vi "Act_LabView3_Task1_jones6sv.vi"() -> ()   [LabVIEW 2016]
uses:
  <vilib>/express/express arith-compare/Formula/XNode/ExpressFormulaBlockNode.xnode
panel:
  out "Numeric":dbl
  in  "Upper limit":dbl
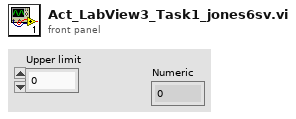
[diagram p1: front panel]
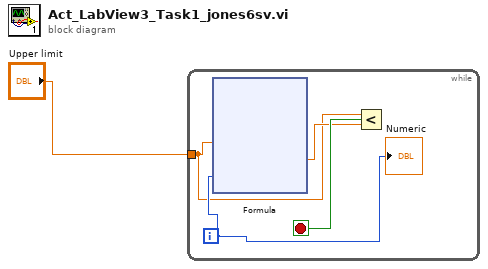
[diagram p0: block diagram]
diagram:
  n1 = while {
    tunnel: "Upper limit" -> [w2]
    i -> [w4]
    stop <- w5 stop-if-true
    n2 = xnode "Formula"("X1"=w2, "X2"=w4) -> ("Result"=w3:dbl)  [unwired: 1 in, 1 out]
    n3 = Less?(x=w2, y=w3) -> (x < y?=w5:bool)
    "Numeric" <- w4
  }
